vi "ROI 2 INI Section.vi"(8 "error in (no error)":errorcluster, 10 "ROI Descriptor":T2 {"Contours"."Type" items=["No Selection", "Point", "Line", "Rectangle", "Oval", "Polygon", "Freehand Region", "Annulus", "Unused2", "Unused3", "Broken Line", "Freehand Line", "Rotated Rectangle"]}, 11 "refnum in":T1) -> (0 "error out":errorcluster, 3 "refnum out":T1)   [LabVIEW 2009]
uses:
  <vilib>/Utility/config.llb/Config Data RefNum.ctl
  <vilib>/Utility/config.llb/Write Key (I32).vi
  <vilib>/Utility/config.llb/Write Key (U32).vi
  <vilib>/Utility/config.llb/NI_LVConfig.lvlib
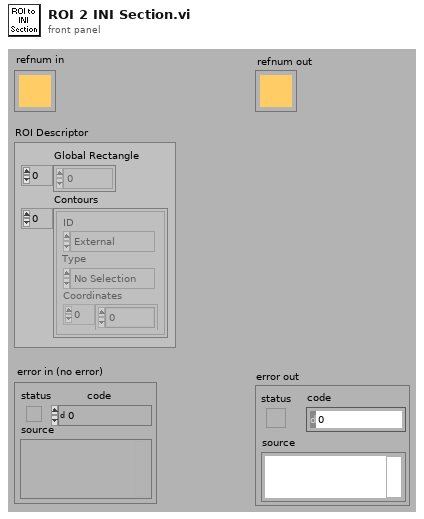
[diagram p1: front panel]
types:
  T1 = typedef "NI_LVConfig.lvlib/Config Data RefNum.ctl" = refnum<k1>
  T2 = typedef "ROI Descriptor" = cluster{"Global Rectangle":i32[], "Contours":cluster{"ID":enum32{"External", "Internal"}, "Type":u32, "Coordinates":i32[]}[]}
  T3 = cluster{"ID":enum32{"External", "Internal"}, "Type":u32, "Coordinates":i32[]}[]
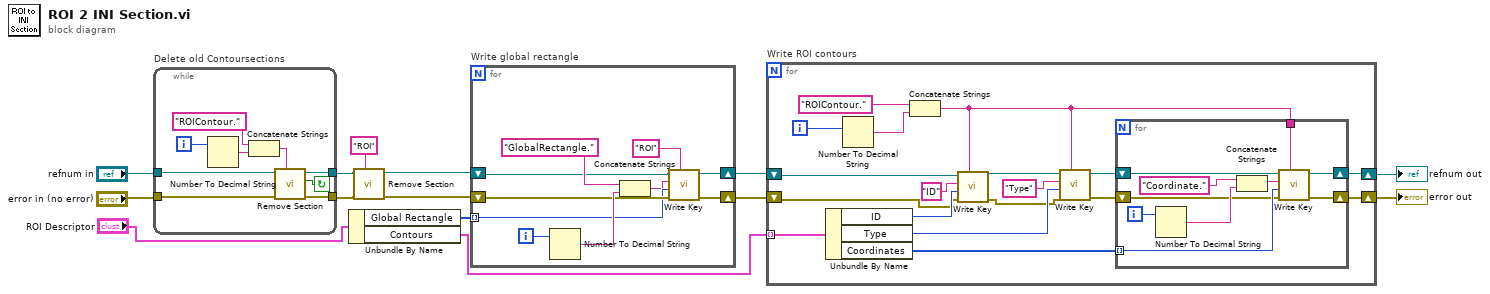
[diagram p0: block diagram]
diagram:
  n1 = while "Delete old Contoursections" {
    tunnel: "refnum in" -> [w23]
    tunnel: "error in (no error)" -> [w22]
    tunnel: [w21] -> w5
    tunnel: [w20] -> w4
    i -> [w16]
    stop <- w19 continue-if-true
    n2 = Number To Decimal String(number=w16) -> (decimal integer string=w18:string)  [unwired: 1 in]
    n3 = Concatenate Strings("ROIContour." ("section"), w18) -> (w15:string)
    n4 = call <vilib>:"Remove Section.vi"("section"=w15, "error in (no error)"=w22, "refnum"=w23) -> ("error out"=w20:errorcluster, "section exists?"=w19:bool, "refnum out"=w21:T1)  [unwired: 6 in]
  }
  n5 = Unbundle By Name("ROI Descriptor") -> ("Global Rectangle"=w9:i32[], "Contours"=w13:T3)
  n6 = call <vilib>:"Remove Section.vi"("section"="ROI", "error in (no error)"=w4, "refnum"=w5) -> ("error out"=w2:errorcluster, "refnum out"=w3:T1)  [unwired: 6 in, 1 out]
  n7 = for "Write global rectangle" {
    shift-right: [w28] -> w8
    shift-left: w2 -> [w29]
    shift-right: [w26] -> w10
    shift-left: w3 -> [w27]
    tunnel: w9 -> [w25] mode=indexing
    i -> [w31]
    n8 = Number To Decimal String(number=w31) -> (decimal integer string=w32:string)  [unwired: 1 in]
    n9 = Concatenate Strings("GlobalRectangle." ("section"), w32) -> (w24:string)
    n10 = call-poly <vilib>:"Write Key.vi"("section"="ROI", "error in (no error)"=w29, "value"=w25, "key"=w24, "refnum"=w27) -> ("error out"=w28:errorcluster, "refnum out"=w26:T1)  [unwired: 4 in, 1 out]
  }
  n11 = for "Write ROI contours" {
    tunnel: w13 -> [w51] mode=indexing
    shift-right: [w35] -> w11
    shift-left: w10 -> [w46]
    shift-right: [w34] -> w12
    shift-left: w8 -> [w36]
    i -> [w48]
    n12 = Unbundle By Name(w51) -> ("ID"=w45:enum32{"External", "Internal"}, "Type"=w41:u32, "Coordinates"=w50:i32[])
    n13 = Number To Decimal String(number=w48) -> (decimal integer string=w47:string)  [unwired: 1 in]
    n14 = Concatenate Strings("ROIContour." ("section"), w47) -> (w38:string)
    n15 = call-poly <vilib>:"Write Key.vi"("section"=w38, "error in (no error)"=w36, "value"=w45, "key"="ID", "refnum"=w46) -> ("error out"=w40:errorcluster, "refnum out"=w43:T1)  [unwired: 4 in, 1 out]
    n16 = call-poly <vilib>:"Write Key.vi"("section"=w38, "error in (no error)"=w40, "value"=w41, "key"="Type", "refnum"=w43) -> ("error out"=w37:errorcluster, "refnum out"=w39:T1)  [unwired: 4 in, 1 out]
    n17 = for {
      tunnel: w50 -> [w56] mode=indexing
      tunnel: w38 -> [w60]
      shift-right: [w54] -> w34
      shift-left: w37 -> [w55]
      shift-right: [w53] -> w35
      shift-left: w39 -> [w61]
      i -> [w59]
      n18 = Number To Decimal String(number=w59) -> (decimal integer string=w58:string)  [unwired: 1 in]
      n19 = Concatenate Strings("Coordinate." ("string"), w58) -> (w57:string)
      n20 = call-poly <vilib>:"Write Key.vi"("section"=w60, "error in (no error)"=w55, "value"=w56, "key"=w57, "refnum"=w61) -> ("error out"=w54:errorcluster, "refnum out"=w53:T1)  [unwired: 4 in, 1 out]
    }
  }
  "error out" <- w12
  "refnum out" <- w11
